vi "Read Module NVMEM.vi"(8 "error in":errorcluster, 11 "slsc module":refnum<k21>) -> (0 "error out":errorcluster, 1 "slot number":u32, 2 "switches json":string, 3 "product name":string)   [LabVIEW 2017, in "SLSC Switch Scripting.lvlib"]
uses:
  SLSC Switch Scripting.lvlib
  <vilib>/SLSC/Initialize Session with Devices.vi
  <vilib>/SLSC/Close Session.vi
  <resource>/objmgr/slsc.rc
  <vilib>/SLSC/SLSC.lvlib
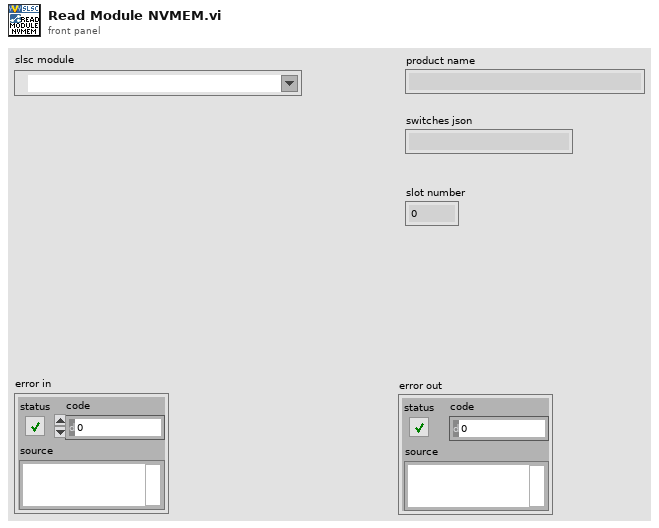
[diagram p1: front panel]
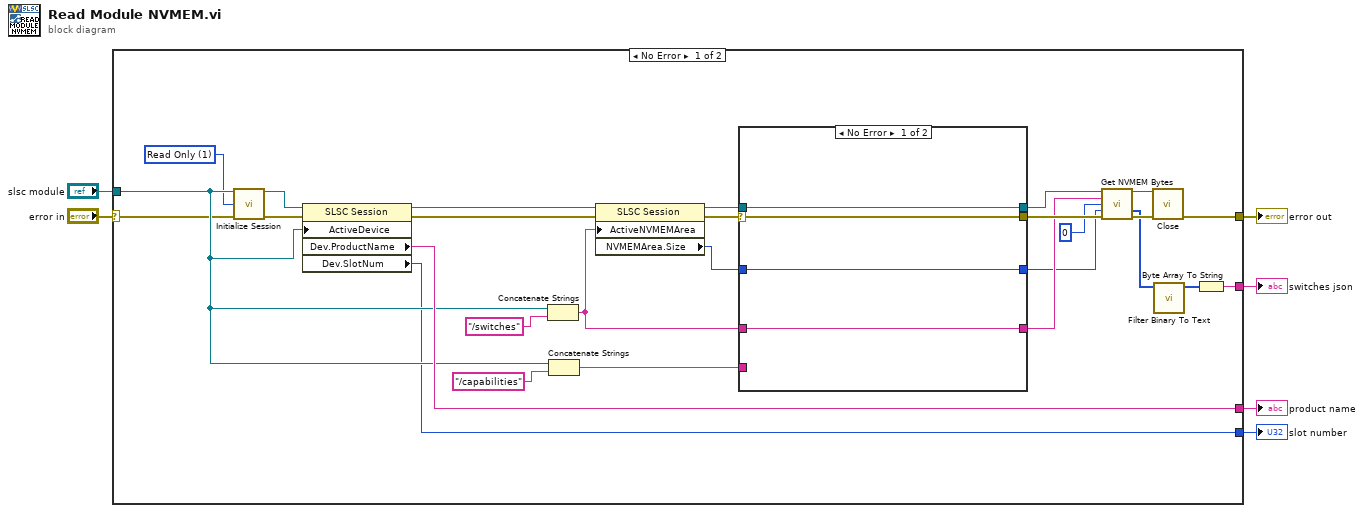
[diagram p0: block diagram]
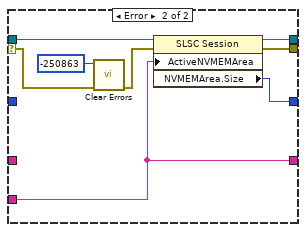
[diagram p2: hidden frame]
diagram:
  n1 = case shown="No Error" "error in" {
    selector: "error in" -> [w12 w46]
    tunnel: [w31 _] -> w6
    tunnel: "slsc module" -> [w25 _]
    tunnel: [w13 _] -> w4
    tunnel: [w11 _] -> w2
    tunnel: [w10 w46] -> w1
    frame No Error {
      w7 = 1 items=["None"=0, "Read Only"=1, "Read/Write"=3] ("reservation access (Read/Write)")
      n2 = call-poly <vilib>:"Initialize Session.vi"("devices"=w25, "reservation access (Read/Write)"=w7, "error in (no error)"=w12) -> ("session out"=w33:refnum<k21>, "error out"=w32:errorcluster)  [unwired: 11 in]
      n3 = property class="SLSC Session"(reference=w33, error in=w32, "ActiveDevice"=w25) -> (reference out=w30:refnum<k21>, error out=w27:errorcluster, "Dev.ProductName"=w31:string, "Dev.SlotNum"=w11:u32)
      n4 = Concatenate Strings(w25, "/switches" ("string")) -> (w21:string)
      n5 = Concatenate Strings(w25, "/capabilities" ("string")) -> (w23:string)
      n6 = property class="SLSC Session"(reference=w30, error in=w27, "ActiveNVMEMArea"=w21) -> (reference out=w24:refnum<k21>, error out=w28:errorcluster, "NVMEMArea.Size"=w22:u32)
      n7 = case shown="No Error" w28 {
        selector: w28 -> [w34 w40]
        tunnel: w24 -> [w35 w45]
        tunnel: w23 -> [_ w43]
        tunnel: w22 -> [w36 _]
        tunnel: [w36 w44] -> w16
        tunnel: w21 -> [w37 _]
        tunnel: [w37 w43] -> w18
        tunnel: [w35 w42] -> w20
        tunnel: [w34 w41] -> w19
        frame No Error {
        }
        frame Error {
          n8 = call <vilib>:"Clear Errors.vi"("error in (no error)"=w40, "specific error code to clear (0: all)"=-250863) -> ("error out"=w39:errorcluster)  [unwired: 4 in, 1 out]
          n9 = property class="SLSC Session"(reference=w45, error in=w39, "ActiveNVMEMArea"=w43) -> (reference out=w42:refnum<k21>, error out=w41:errorcluster, "NVMEMArea.Size"=w44:u32)
        }
      }
      n10 = call <vilib>:"Get NVMEM Bytes.vi"("session in"=w20, "NVMEM area"=w18, "data address"=u32 0, "data size"=w16, "error in (no error)"=w19) -> ("session out"=w15:refnum<k21>, "data out"=w8:u8[], "error out"=w14:errorcluster)  [unwired: 6 in, 2 out]
      n11 = call-poly <vilib>:"Close.vi"("session in"=w15, "error in (no error)"=w14) -> ("error out"=w10:errorcluster)  [unwired: 13 in]
      n12 = call "Filter Binary To Text.vi"("raw input"=w8) -> ("filtered output"=w9:u8[])  [unwired: 10 in]
      n13 = Byte Array To String(unsigned byte array=w9) -> (string=w13:string)
    }
    frame Error {
    }
  }
  "product name" <- w6
  "switches json" <- w4
  "error out" <- w1
  "slot number" <- w2
